vi "Choreo_TrajectoryDifferential_Equals.vi"(9 "otherChoreoTrajectoryDifferential":T1, 11 "ChoreoTrajectoryDifferential":T1) -> (3 "equal":bool)   [LabVIEW 2019, in "ChoreoLib.lvlib"]
doc: "Determine if two trajectories are equal\n\nInputs: \n - ChoreoTrajectory - cluster - Input trajectory\n - Other ChoreoTrajectory - cluster - Trajectory to compare\n\nOutputs:\n - Equals - boolean - TRUE if trajectories are equal."
uses:
  ChoreoLib.lvlib
  TypeDef/ChoreoTrajectoryDifferential.ctl
  TypeDef/ChoreoDifferentialSample.ctl
  TypeDef/ChoreoEventMarker.ctl
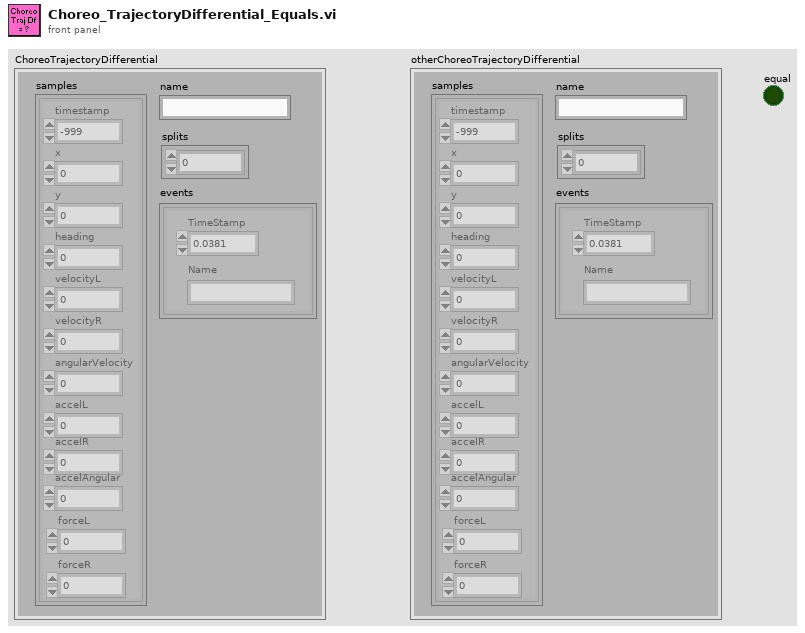
[diagram p1: front panel]
types:
  T1 = typedef "ChoreoLib.lvlib/ChoreoTrajectoryDifferential.ctl" = cluster{"name":string, "samples":T2[], "splits":i32[], "events":T3[]}
  T2 = typedef "ChoreoLib.lvlib/ChoreoDifferentialSample.ctl" = cluster{"timestamp":dbl, "x":dbl, "y":dbl, "heading":dbl, "velocityL":dbl, "velocityR":dbl, "angularVelocity":dbl, "accelL":dbl, "accelR":dbl, "accelAngular":dbl, "forceL":dbl, "forceR":dbl}
  T3 = typedef "ChoreoLib.lvlib/ChoreoEventMarker.ctl" = cluster{"TimeStamp":dbl, "Name":string}
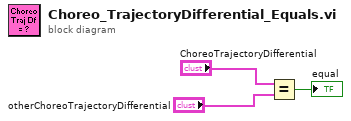
[diagram p0: block diagram]
diagram:
  n1 = Equal?(x="ChoreoTrajectoryDifferential", y="otherChoreoTrajectoryDifferential") -> (x = y?=→"equal":bool)
